vi "flattenAngularVelocityToXML.vi"   [LabVIEW 2012, in "UnitsAndXML.lvlib"]
doc: "Generates an XML string for <B>angularVelocity</B> in the unit specified in <B>angularVelocityUnitInXML</B>. Connect <B>angularVelocity</B> and <B>angularVelocityAgain</B> to the same source. The VI uses <B>angularVelocityAgain</B> to obtain the data name."
uses:
  <userlib>/Common/UnitsAndXML/UnitsAndXML.lvlib
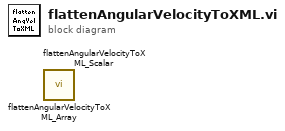
[diagram p0: block diagram]
diagram:
  n1 = call <userlib>:"flattenAngularVelocityToXML_Array.vi"() -> ()  [unwired: 10 in, 2 out]
  n2 = call <userlib>:"flattenAngularVelocityToXML_Scalar.vi"() -> ()  [unwired: 10 in, 2 out]
